vi "Clear Macro Data.vi"(11 "Macro":T1) -> (3 "Macro out":T1)   [LabVIEW 2020, in "MacroAssert.lvlib"]
doc: "Clears <B>Macro</B> in preparation to create a new macro with some starting information."
uses:
  MacroAssert.lvlib
  CTLs/Macro Cluster V3.ctl
  CTLs/Macro Config V3.ctl
  CTLs/Step V3.ctl
  CTLs/Step Type V3.ctl
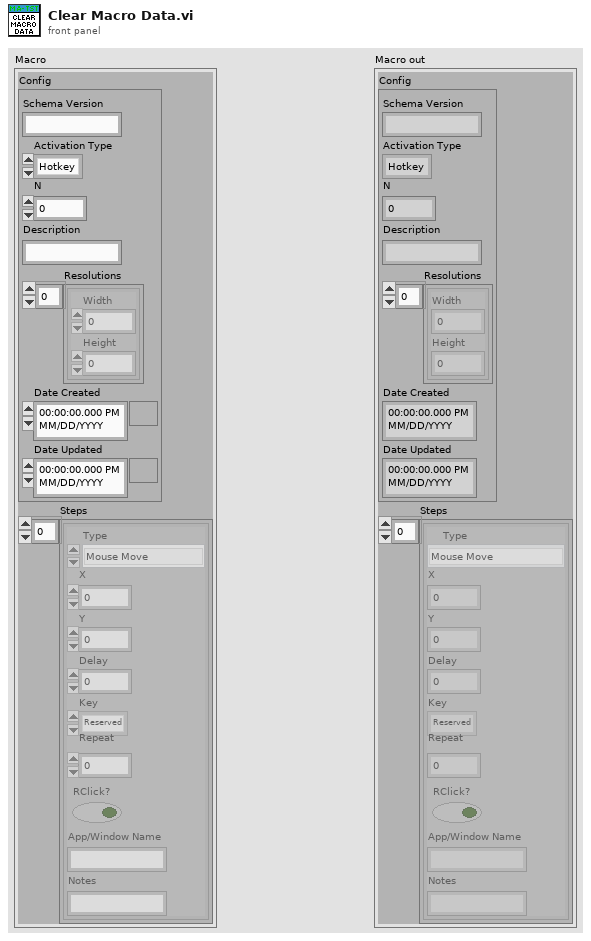
[diagram p1: front panel]
types:
  T1 = typedef "MacroAssert.lvlib/Macro Cluster V3.ctl" = cluster{"Config":T2, "Steps":T3[]}
  T2 = typedef "MacroAssert.lvlib/Macro Config V3.ctl" = cluster{"Schema Version":string, "Activation Type":enum32{"Hotkey", "Automatic"}, "N":i32, "Description":string, "Resolutions":cluster{"Width":i16, "Height":i16}[], "Date Created":timestamp, "Date Updated":timestamp}
  T3 = typedef "MacroAssert.lvlib/Step V3.ctl" = cluster{"Type":T4, "X":i32, "Y":i32, "Delay":i32, "Key":u8, "Repeat":i32, "RClick?":bool, "App/Window Name":string, "Notes":string}
  T4 = typedef "MacroAssert.lvlib/Step Type V3.ctl" = enum16{"Mouse Move", "Mouse Click", "Key Press", "Wait", "Mouse Down", "Mouse Up", "Key Down", "Key Up", "Run Application", "Maximize Window", "Restore Window", "Minimize Window", "Close Window", "Bring Window to Front", "Send Window to Back"}
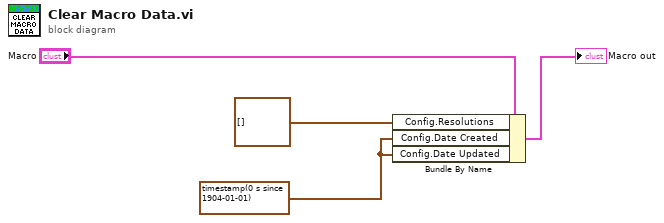
[diagram p0: block diagram]
diagram:
  w1 = timestamp(0 s since 1904-01-01) ("Date Created")
  n1 = Bundle By Name(cluster="Macro", "Config.Resolutions"=cluster{"Width":i16, "Height":i16}[] [] ("Resolutions"), "Config.Date Created"=w1, "Config.Date Updated"=w1) -> (→"Macro out":T1)
